vi "Acc2.vi"() -> ()   [LabVIEW 2020]
uses:
  <vilib>/Analysis/NI_AAL_SigProc.lvlib
panel:
  out "width":i32=3
  out "threshold 2":dbl=-0.12
  out "threshold":dbl=-0.12
  out "?":dynamicdata(graph)
  out "?":dynamicdata(graph)
  out "?":dynamicdata(graph)
  in  "Motor Trottle":dbl(slide) scale=0.0..5.0
  out "Selected Signals":dynamicdata(graph)
  out "Signal Filtered":dynamicdata(graph)
  out "Motor":bool
  in  "Motor Enable":bool
  out "Swing":bool
  out "Heel Strike 2":bool
  out "Heel Strike 1":bool
  in  "Record Signal":bool
  in  "STOP":bool
  # "Gait Events"
  # "Preak Detector Parameters"
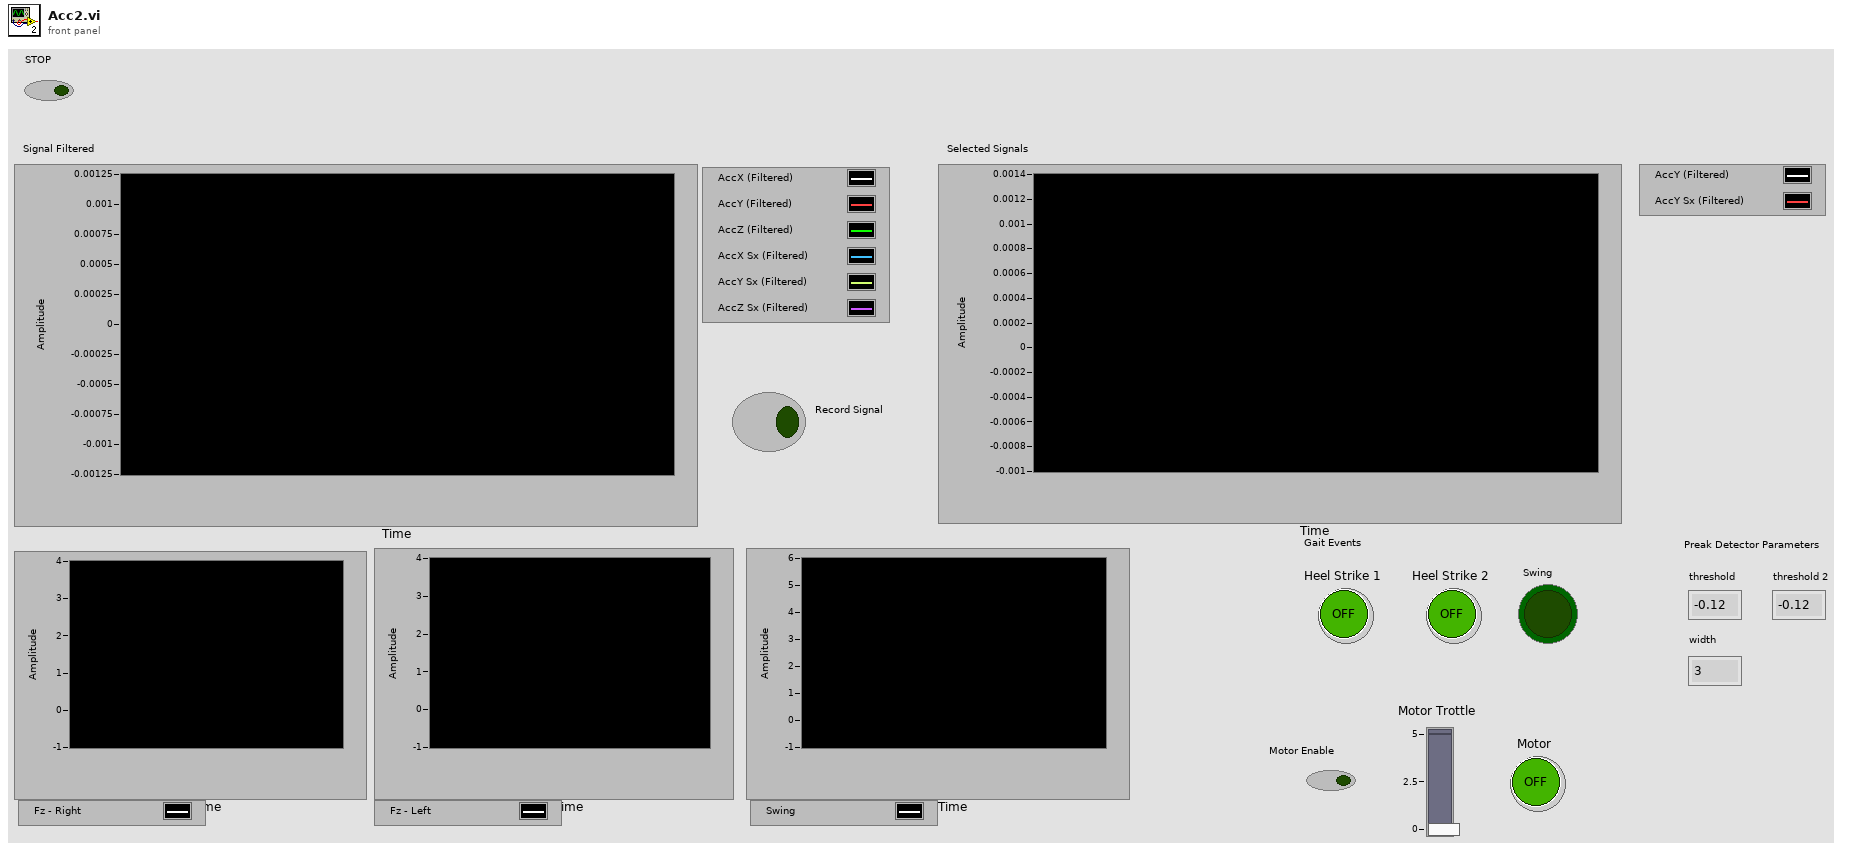
[diagram p1: front panel]
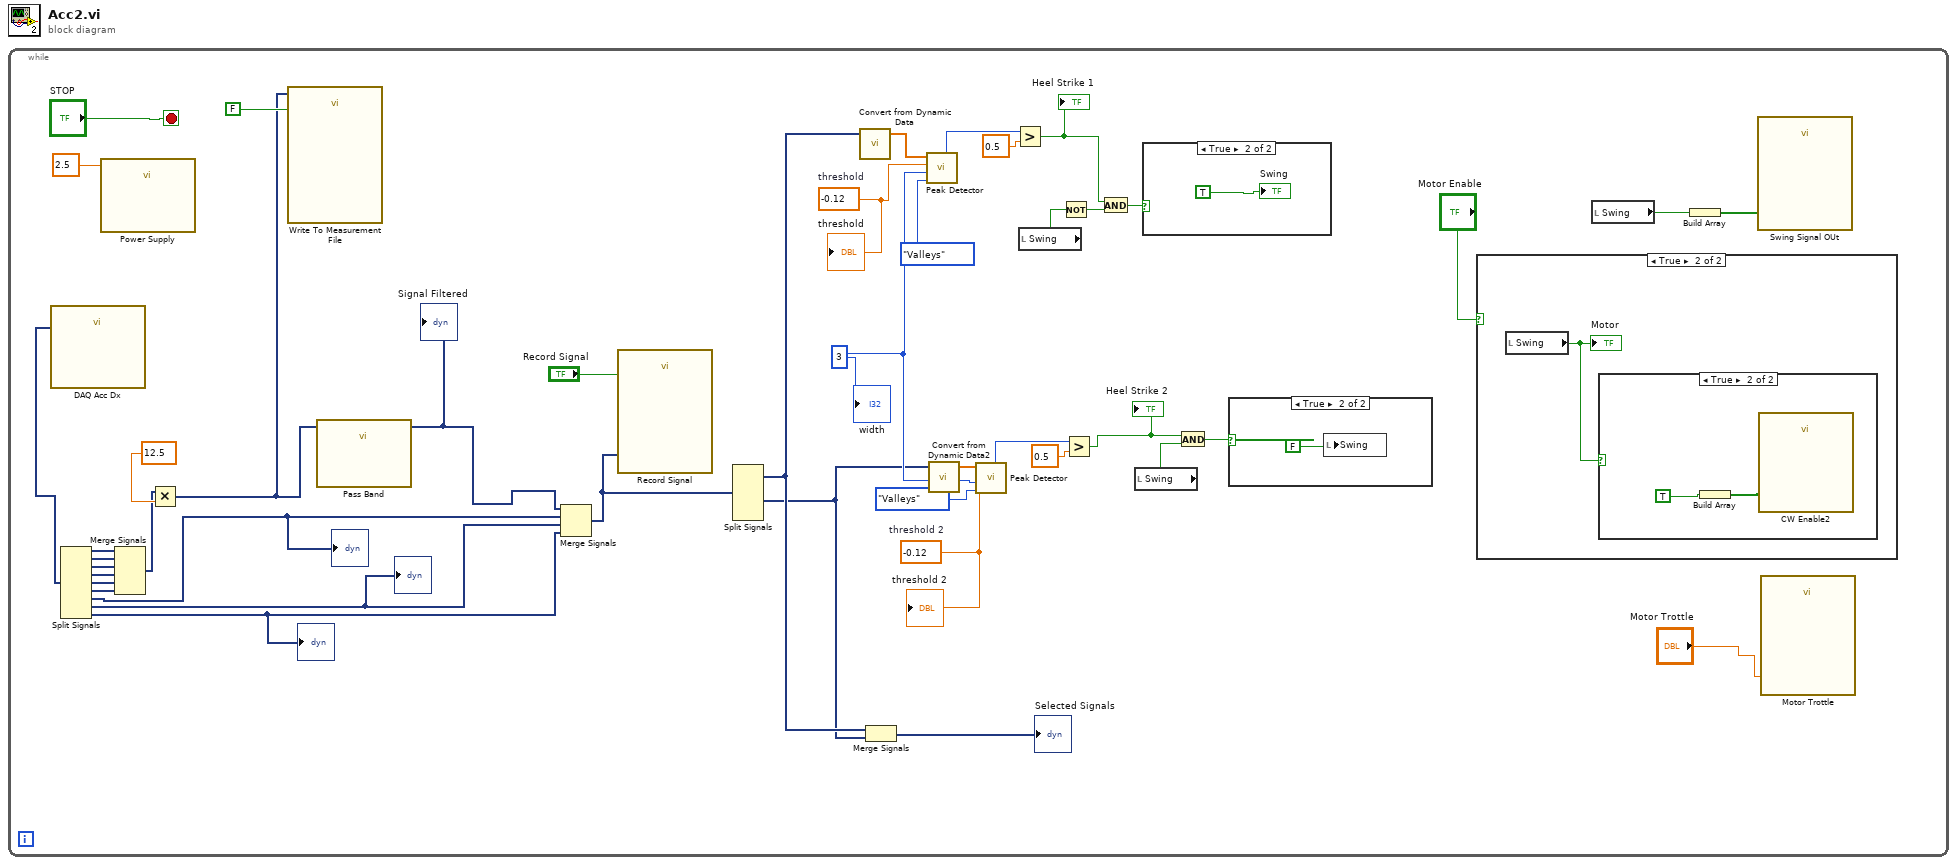
[diagram p0: block diagram]
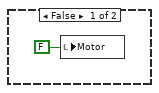
[diagram p2: hidden frame]
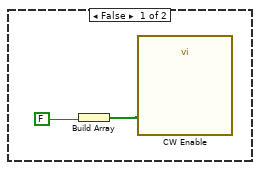
[diagram p3: hidden frame]
diagram:
  n1 = while {
    stop <- "STOP" stop-if-true
    w10 = -0.12  # threshold
    w11 = -0.12  # threshold 2
    w12 = 3 ("width")
    n2 = call "DAQ Acc Dx"() -> ("data"=w20:dynamicdata)  [unwired: 16 in, 3 out]
    n3 = Split Signals(w20) -> (w19:dynamicdata, w18:dynamicdata, w17:dynamicdata, w16:dynamicdata, w15:dynamicdata, w14:dynamicdata, w3:dynamicdata, w2:dynamicdata, w1:dynamicdata)  [unwired: 9 in]
    "?" <- w3
    "?" <- w2
    "?" <- w1
    n4 = call "Power Supply"("data"=2.5) -> ()  [unwired: 17 in, 2 out]
    n5 = Merge Signals(w19, w18, w17, w16, w15, w14) -> (w13:dynamicdata)
    n6 = Multiply(x=w13, y=12.5) -> (x*y=w21:dynamicdata)
    n7 = call "Write To Measurement File"("Signals"=w21, "Enable"=FALSE) -> ()  [unwired: 15 in, 3 out]
    n8 = call "Pass Band"("Signal"=w21) -> ("Filtered Signal"=w24:dynamicdata)  [unwired: 9 in, 1 out]
    "Signal Filtered" <- w24
    n9 = Merge Signals(w24, w3, w2, w1) -> (w23:dynamicdata)
    n10 = call "Record Signal"("Signals"=w23, "Enable"="Record Signal") -> ()  [unwired: 15 in, 3 out]
    n11 = Split Signals(w23) -> (w5:dynamicdata, w4:dynamicdata)  [unwired: 7 in, 5 out]
    n12 = call "Convert from Dynamic Data"("Dynamic Data Type"=w5) -> ("Array"=w36:dbl[])  [unwired: 3 in]
    n13 = Merge Signals(w5, w4) -> (→"Selected Signals":dynamicdata)
    n14 = call <vilib>:"Peak Detector.vi"("peaks/valleys"=enum32{"Peaks", "Valleys"}."Valleys", "width"=w12, "threshold"=w10, "X"=w36) -> ("# found"=w34:i32)  [unwired: 3 in, 4 out]
    n15 = call "Convert from Dynamic Data2"("Dynamic Data Type"=w4) -> ("Array"=w29:dbl[])  [unwired: 3 in]
    n16 = call <vilib>:"Peak Detector.vi"("peaks/valleys"=enum32{"Peaks", "Valleys"}."Valleys", "width"=w12, "threshold"=w11, "X"=w29) -> ("# found"=w32:i32)  [unwired: 3 in, 4 out]
    n17 = Greater?(x=w34, y=0.5) -> (0:w7:bool)
    "Heel Strike 1" <- w7
    n18 = local read "Swing"() -> (w9:bool)
    n19 = Not(x=w9) -> (.not. x?=w6:bool)
    n20 = Greater?(x=w32, y=0.5) -> (0:w30:bool)
    "Heel Strike 2" <- w30
    n21 = And(x=w7, y=w6) -> (x .and. y?=w8:bool)
    n22 = local read "Swing"() -> (w38:bool)
    n23 = case shown="True" w8 {
      frame False {
      }
      frame True {
        "Swing" <- TRUE
      }
    }
    n24 = And(x=w30, y=w38) -> (x .and. y?=w39:bool)
    n25 = case shown="True" w39 {
      frame False {
      }
      frame True {
        n26 = local write "Swing"(FALSE) -> ()
      }
    }
    n27 = case shown="True" "Motor Enable" {
      frame False {
        n28 = local write "Motor"(FALSE) -> ()
      }
      frame True {
        n29 = local read "Swing"() -> (w46:bool)
        "Motor" <- w46
        n30 = case shown="True" w46 {
          frame False {
            n31 = Build Array(FALSE) -> (w48:bool[])
            n32 = call "CW Enable"("data"=w48) -> ()  [unwired: 17 in, 2 out]
          }
          frame True {
            n33 = Build Array "Build Array"(TRUE) -> (w49:bool[])
            n34 = call "CW Enable2"("data"=w49) -> ()  [unwired: 17 in, 2 out]
          }
        }
      }
    }
    n35 = local read "Swing"() -> (w26:bool)
    n36 = Build Array "Build Array"(w26) -> (w25:bool[])
    n37 = call "Swing Signal OUt"("data"=w25) -> ()  [unwired: 17 in, 2 out]
    n38 = call "Motor Trottle"("data"="Motor Trottle") -> ()  [unwired: 17 in, 2 out]
    "threshold" <- w10
    "threshold 2" <- w11
    "width" <- w12
  }
